vi "Inverse f Noise Waveform.vi"(0 "noise density":dbl=0.1 format="%.2p", 1 "reset signal (F)":bool, 5 "exponent":dbl=1.0 format="%.2p", 7 "filter specifications":T3={"lower cutoff freq"=0.1, "higher cutoff freq"=100.0, "order"=5} {"higher cutoff freq" format="%#_2p"; "lower cutoff freq" format="%#_2p"}, 9 "seed":i32=-1, 11 "error in (no error)":errorcluster, 12 "sampling info":cluster{"Fs":dbl, "#s":dbl}={"Fs"=1000.0, "#s"=1000.0} {"Fs" format="%.2p"}, 13 "reference freq (Hz)":dbl=1.0 format="%.2p") -> (4 "signal out":waveform(dbl), 6 "magnitude error (dB)":T1 {"magnitude (dB)" format="%.2p"; "frequency (Hz)" format="%.2p"}, 8 "expected rms":dbl=1.0 format="%.2p", 10 "filter information":T2, 15 "error out":errorcluster)   [LabVIEW 2020, in "NI_MABase.lvlib"]
doc: "Generates a continuous noise waveform with a power spectral density that is inversely proportional to frequency over a specified frequency range."
uses:
  NI_MABase.lvlib
  NI_AALBase.lvlib
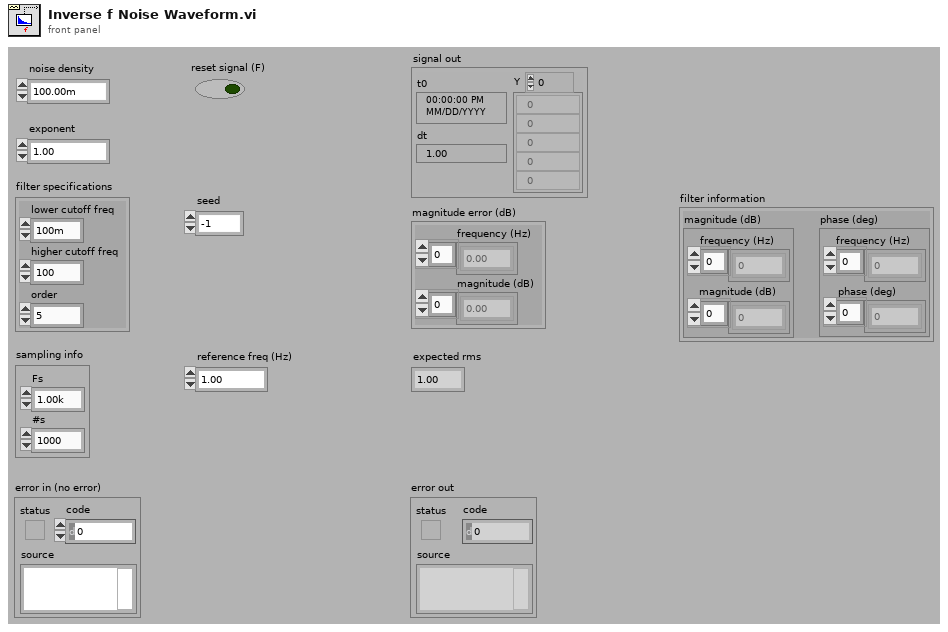
[diagram p1: front panel]
types:
  T1 = cluster{"frequency (Hz)":dbl[], "magnitude (dB)":dbl[]}
  T2 = cluster{"magnitude (dB)":cluster{"frequency (Hz)":dbl[], "magnitude (dB)":dbl[]}, "phase (deg)":cluster{"frequency (Hz)":dbl[], "phase (deg)":dbl[]}}
  T3 = cluster{"lower cutoff freq":dbl, "higher cutoff freq":dbl, "order":i32}
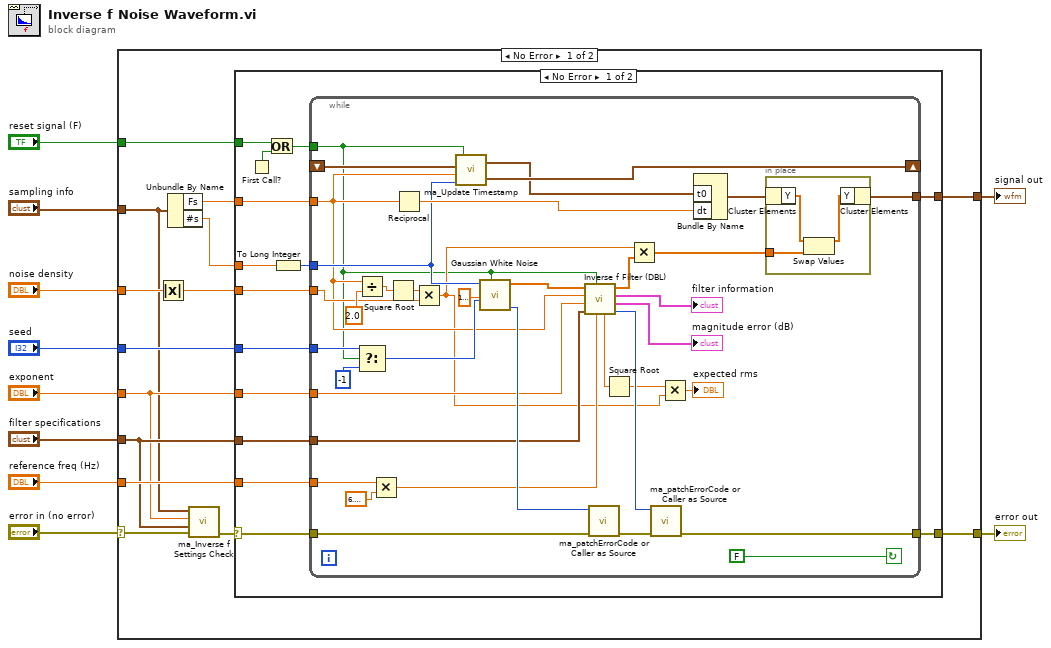
[diagram p0: block diagram]
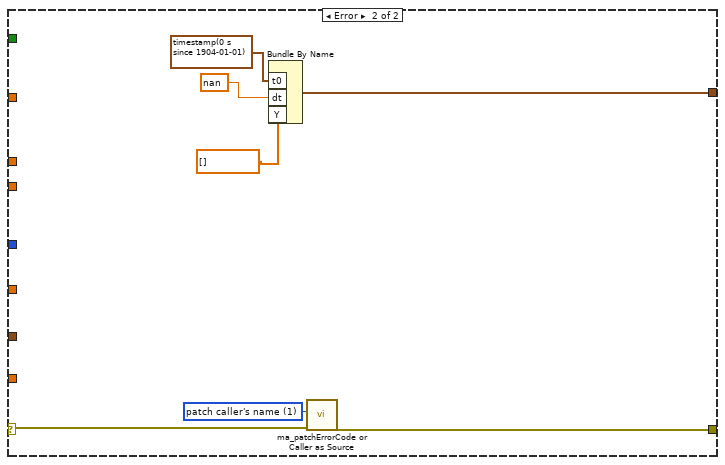
[diagram p2: hidden frame]
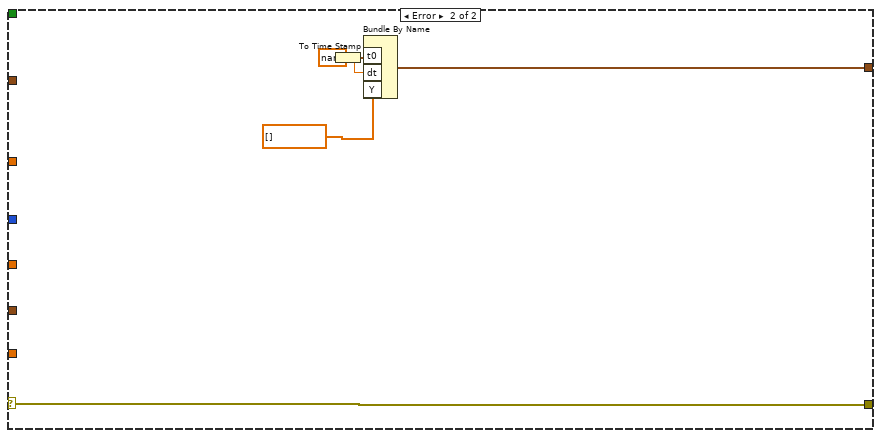
[diagram p3: hidden frame]
diagram:
  n1 = case shown="No Error" "error in (no error)" {
    selector: "error in (no error)" -> [w16 w90]
    tunnel: [w19 w90] -> w10
    tunnel: "sampling info" -> [w12 _]
    tunnel: [w22 w89] -> w8
    tunnel: "noise density" -> [w24 _]
    tunnel: "seed" -> [w23 _]
    tunnel: "exponent" -> [w13 _]
    tunnel: "filter specifications" -> [w14 _]
    tunnel: "reference freq (Hz)" -> [w18 _]
    tunnel: "reset signal (F)" -> [w11 _]
    frame No Error {
      n2 = Absolute Value(x=w24) -> (abs(x)=w17:dbl)
      n3 = Unbundle By Name(w12) -> ("Fs"=w21:dbl, "#s"=w20:dbl)
      n4 = call "ma_Inverse f Settings Check.vi"("error in (no error)"=w16, "filter specifications"=w14, "exponent"=w13, "sampling info"=w12) -> ("error out"=w15:errorcluster)  [unwired: 1 in, 6 out]
      n5 = case shown="No Error" w15 {
        selector: w15 -> [w28 w79]
        tunnel: w17 -> [w38 _]
        tunnel: w23 -> [w37 _]
        tunnel: [w36 w83] -> w22
        tunnel: [w30 w81] -> w19
        tunnel: w21 -> [w35 _]
        tunnel: w20 -> [w34 _]
        tunnel: w13 -> [w32 _]
        tunnel: w14 -> [w31 _]
        tunnel: w18 -> [w29 _]
        tunnel: w11 -> [w25 _]
        frame No Error {
          n6 = First Call?() -> (First Call?: T/F=w27:bool)
          n7 = Or(x=w25, y=w27) -> (x .or. y?=w26:bool)
          n8 = To Long Integer(number=w34) -> (32bit integer=w33:i32)
          n9 = while {
            tunnel: w33 -> [w69]
            tunnel: w35 -> [w46]
            tunnel: [w41] -> w36
            shift-left: _ -> [w61]
            shift-right: [w63] -> _
            tunnel: w37 -> [w75]
            tunnel: w26 -> [w39]
            tunnel: w38 -> [w48]
            tunnel: w32 -> [w45]
            tunnel: w31 -> [w64]
            tunnel: [w68] -> w30
            tunnel: w28 -> [w65]
            tunnel: w29 -> [w54]
            stop <- FALSE continue-if-true
            n10 = Divide(x=w46, y=2.0) -> (x/y=w56:dbl)
            n11 = Select(t=w75, s=w39, f=-1) -> (s? t:f=w74:i32)
            n12 = Multiply(x=w54, y=6.283185307179586) -> (x*y=w52:dbl)
            n13 = Square Root(x=w56) -> (sqrt(x)=w57:dbl)
            n14 = Reciprocal(x=w46) -> (1/x=w73:dbl)
            n15 = Multiply(x=w57, y=w48) -> (x*y=w43:dbl)
            n16 = call "ma_Update Timestamp.vi"("samples"=w69, "Sampling Rate (Hz)"=w46, "tf previous"=w61, "Reset Generation"=w39) -> ("tf new"=w63:timestamp, "t0"=w62:timestamp)
            n17 = call "Gaussian White Noise.vi"("initialize?"=w39, "seed"=w74, "standard deviation"=1.0000000000000002, "samples"=w69) -> ("error"=w66:i32, "Gaussian noise pattern"=w70:dbl[])  [unwired: 6 in]
            n18 = call "Inverse f Filter (DBL).vi"("unity gain freq (rad/s)"=w52, "reset"=w39, "filter specifications"=w64, "exponent"=w45, "fs"=w46, "X"=w70) -> ("error"=w60:i32, "magnitude error (dB)"=→"magnitude error (dB)":T1, "filter information"=→"filter information":T2, "Filtered X"=w47:dbl[], "noise bandwidth"=w51:dbl)  [unwired: 1 in]
            n19 = call "ma_patchErrorCode or Caller as Source.vi"("error in (no error)"=w65, "error code"=w66) -> ("error out"=w67:errorcluster)  [unwired: 2 in, 7 out]
            n20 = Square Root(x=w51) -> (sqrt(x)=w50:dbl)
            n21 = Multiply(x=w43, y=w47) -> (x*y=w40:dbl[])
            n22 = call "ma_patchErrorCode or Caller as Source.vi"("error in (no error)"=w67, "error code"=w60) -> ("error out"=w68:errorcluster)  [unwired: 2 in, 7 out]
            n23 = Multiply(x=w50, y=w43) -> (x*y=→"expected rms":dbl)
            n24 = Bundle By Name("t0"=w62, "dt"=w73) -> (w42:waveform(dbl))  [unwired: 1 out]
            n25 = in-place {
              in-place-border: w40 -> [w77]
              n26 = in-place-cluster #1(w42) -> ("Y"=w76:dbl[])
              n27 = Swap Values(12:w76, 14:w77) -> (1:w78:dbl[])  [unwired: 1 in, 1 out]
              n28 = in-place-cluster #1("Y"=w78) -> (w41:waveform(dbl))
            }
          }
        }
        frame Error {
          w82 = u16 1 items=["patch error code", "patch caller's name"] ("operation")
          n29 = Bundle By Name("t0"=timestamp(0 s since 1904-01-01), "dt"=nan ("t0"), "Y"=dbl[] []) -> (w83:waveform(dbl))  [unwired: 1 out]
          n30 = call "ma_patchErrorCode or Caller as Source.vi"("error in (no error)"=w79, "operation"=w82) -> ("error out"=w81:errorcluster)  [unwired: 2 in, 7 out]
        }
      }
    }
    frame Error {
      w87 = nan ("t0")
      n31 = To Time Stamp(1:w87) -> (0:w86:timestamp)
      n32 = Bundle By Name("t0"=w86, "dt"=w87, "Y"=dbl[] []) -> (w89:waveform(dbl))  [unwired: 1 out]
    }
  }
  "error out" <- w10
  "signal out" <- w8
